vi "Register Channel.vi"(8 "error in (no error)":errorcluster, 9 "Flow Name":string="default_flow_name", 10 "Channel Config":T2={"name"="", "data_type"=enum."int32", "description"="", "component"="", "unit"="", "bit_field_elements"=[], "enum_types"=[]}, 11 "Sift Client in":refnum<class "Sift Client.lvclass">) -> (0 "error out":errorcluster, 3 "Sift Client out":refnum<class "Sift Client.lvclass">)   [LabVIEW 2024, in "Sift Client.lvlib" / "Sift Client.lvclass"]
doc: "Registers a channel to the specified flow (the default flow is used when none is specified).\n\nCall this for each channel in the flow. Once all channels for a flow have been registered, and all flows created, call Submit Channel Config to send the ingestion config to Sift."
uses:
  Sift Client.lvclass
  Private/Typedefs/Channel Config.ctl
  Types/Data Type.ctl
  Private/Typedefs/Bit Field.ctl
  Private/Typedefs/Enum.ctl
  Private/Typedefs/Flow Config.ctl
  Sift Client.lvclass/Sift Client.ctl
  <vilib>/Utility/miscctls.llb/LVMapReplaceAction.ctl
  Sift Client.lvlib
panel:
  in  "New Flow Config":T1
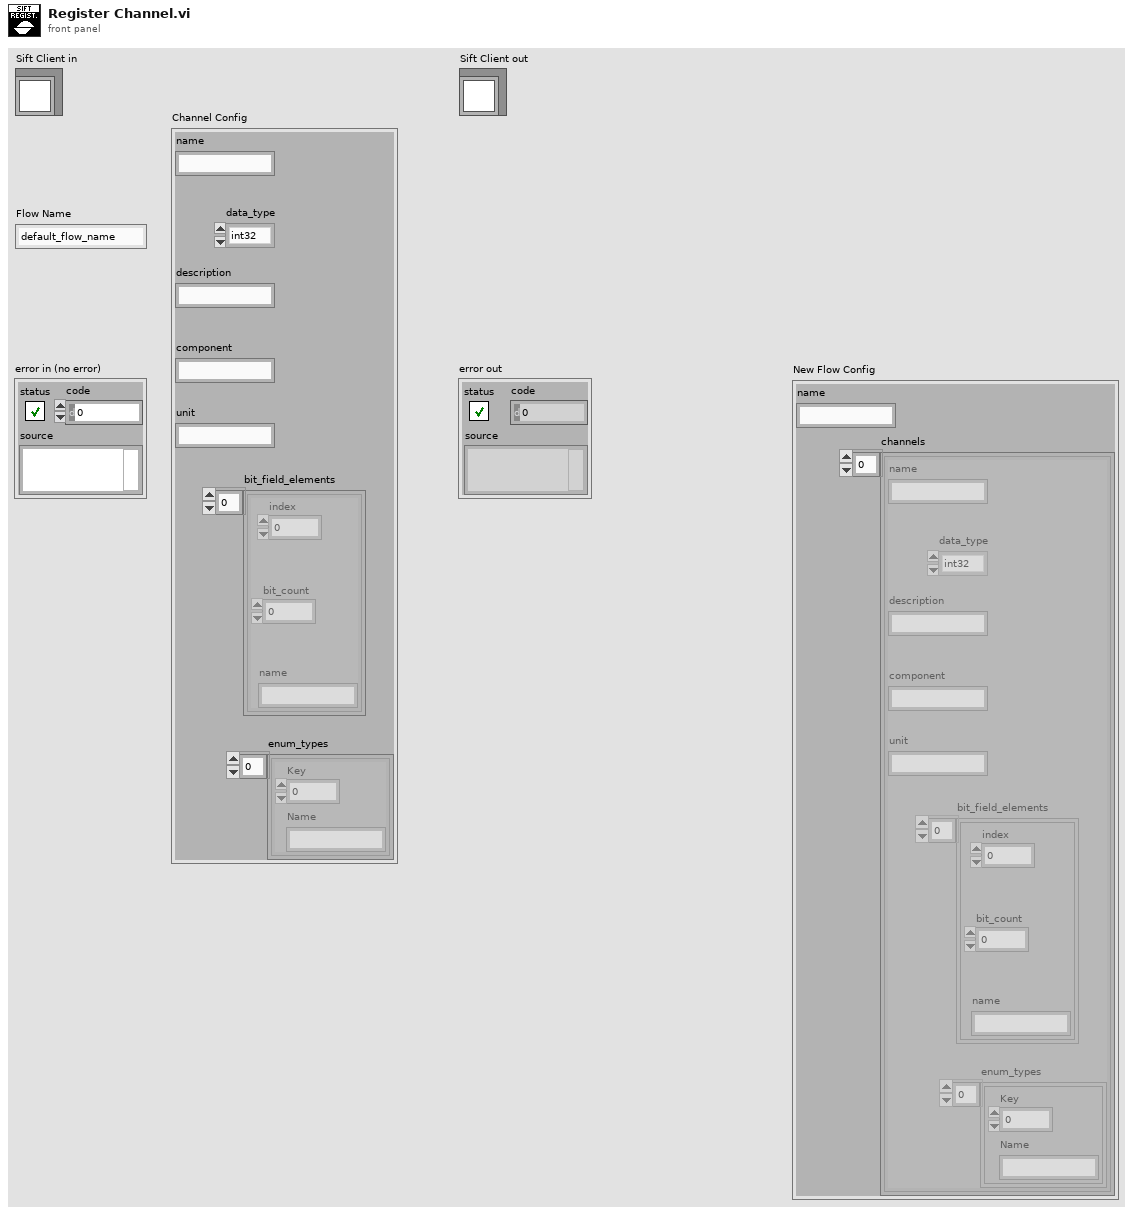
[diagram p1: front panel]
types:
  T1 = typedef "Sift Client.lvlib/Flow Config.ctl" = cluster{"name":string, "channels":T2[]}
  T2 = typedef "Sift Client.lvlib/Channel Config.ctl" = cluster{"name":string, "data_type":T3, "description":string, "component":string, "unit":string, "bit_field_elements":T4[], "enum_types":T5[]}
  T3 = typedef "Sift Client.lvlib/Data Type.ctl" = enum8{"double", "float", "uint64", "int64", "uint32", "int32", "bool", "bit field", "enum"}
  T4 = typedef "Sift Client.lvlib/Bit Field.ctl" = cluster{"index":u32, "bit_count":u32, "name":string}
  T5 = typedef "Sift Client.lvlib/Enum.ctl" = cluster{"Key":u32, "Name":string}
  T6 = typedef "LVMapReplaceAction.ctl" = enum32{"Modify Entry only if found", "Add or Modify Entry", "Delete Entry"}
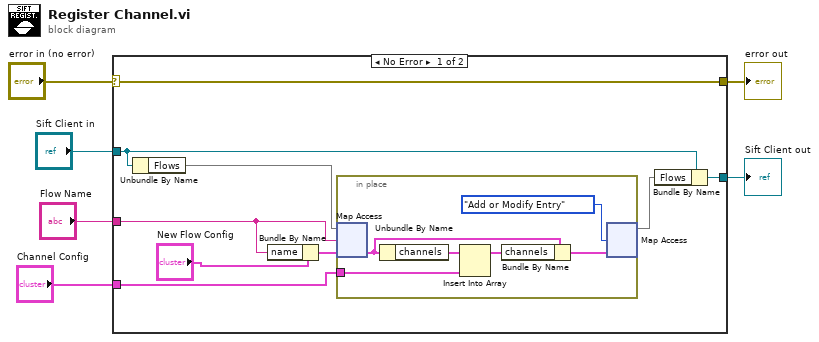
[diagram p0: block diagram]
diagram:
  n1 = case shown="No Error" "error in (no error)" {
    selector: "error in (no error)" -> [w11 w23]
    tunnel: [w11 w23] -> w5
    tunnel: "Sift Client in" -> [w14 w22]
    tunnel: "Channel Config" -> [w12 _]
    tunnel: "Flow Name" -> [w15 _]
    tunnel: [w13 w22] -> w1
    frame No Error {
      n2 = Unbundle By Name(w14) -> ("Flows"=w10:map{string, T1})
      n3 = Bundle By Name(cluster="New Flow Config", "name"=w15) -> (w7:T1)
      n4 = in-place {
        in-place-border: w12 -> [w21]
        n5 = in-place-map #1(w10, w15, w7) -> (w16:T1)  [unwired: 1 out]
        n6 = Unbundle By Name(w16) -> ("channels"=w19:T2[])
        n7 = Insert Into Array(array=w19, new element=w21) -> (w18:T2[])  [unwired: 1 in]
        n8 = Bundle By Name(cluster=w16, "channels"=w18) -> (w17:T1)
        n9 = in-place-map #1(w17, LVMapReplaceAction."Add or Modify Entry" ("action")) -> (w9:map{string, T1})  [unwired: 2 out]
      }
      n10 = Bundle By Name(cluster=w14, "Flows"=w9) -> (w13:refnum<class "Sift Client.lvclass">)
    }
    frame Error {
    }
  }
  "error out" <- w5
  "Sift Client out" <- w1
